vi "New builtInTest.vi"(8 "error in":errorcluster, 11 "core builtInTest configuration (default)":T1) -> (0 "error out":errorcluster, 3 "new builtInTest out":refnum<k24>)   [LabVIEW 2020, in "Ballard_1553_Hardware_ni.lvlib"]
uses:
  Ballard_1553_Hardware_ni.lvlib
  C:/Users/Administrator/Desktop/GIT/Ballard-MIL-STD-1553-Custom-Device/Source/System Explorer/SubVIs/Parse XML Ballard/1.2/BTIXML_SerDes.dll
  Ballard-MIL-STD-1553-Custom-Device/Source/System Explorer/SubVIs/Parse XML Ballard/1.2/BTIXML_SerDes.dll
  _typedefs/core_builtInTests_type.ctl
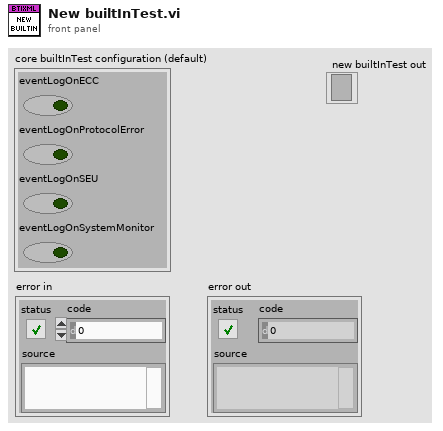
[diagram p1: front panel]
types:
  T1 = typedef "Ballard_1553_Hardware_ni.lvlib/core_builtInTests_type.ctl" = cluster{"eventLogOnECC":bool, "eventLogOnProtocolError":bool, "eventLogOnSEU":bool, "eventLogOnSystemMonitor":bool}
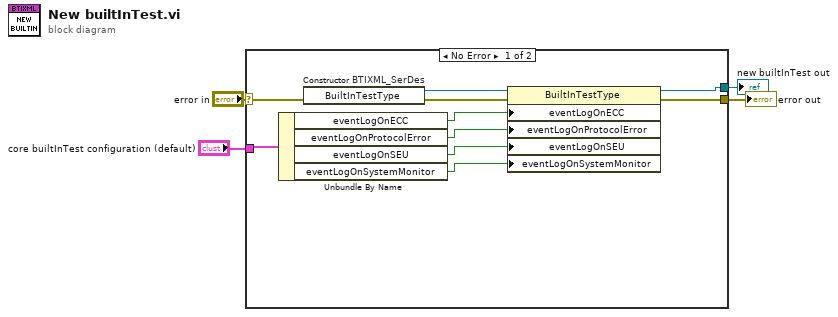
[diagram p0: block diagram]
diagram:
  n1 = case shown="No Error" "error in" {
    selector: "error in" -> [w14 w15]
    tunnel: [w11 w15] -> w3
    tunnel: [w10 _] -> w1
    tunnel: "core builtInTest configuration (default)" -> [w9 _]
    frame No Error {
      n2 = Unbundle By Name(w9) -> ("eventLogOnECC"=w8:bool, "eventLogOnProtocolError"=w7:bool, "eventLogOnSEU"=w6:bool, "eventLogOnSystemMonitor"=w5:bool)
      n3 = constructor on="BTIXML_SerDes" class="BuiltInTestType"(error in=w14) -> (reference out=w13:refnum<k24>, error out=w12:errorcluster)  [unwired: 2 in, 1 out]
      n4 = property class="BuiltInTestType"(reference=w13, error in=w12, "eventLogOnECC"=w8, "eventLogOnProtocolError"=w7, "eventLogOnSEU"=w6, "eventLogOnSystemMonitor"=w5) -> (reference out=w10:refnum<k24>, error out=w11:errorcluster)
    }
    frame Error {
    }
  }
  "error out" <- w3
  "new builtInTest out" <- w1
